vi "整合数据6.vi"(0 "Data in":u8[](array[numeric])) -> (5 "P1":u16, 6 "I1":u16, 7 "D1":u16, 8 "D2":u16, 9 "P2":u16, 10 "I2":u16)   [LabVIEW 2016]
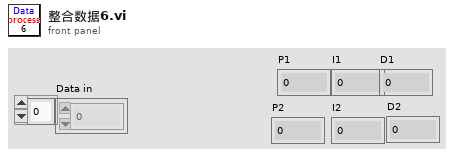
[diagram p1: front panel]
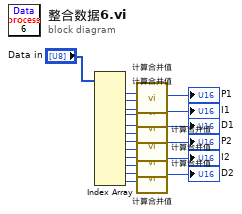
[diagram p0: block diagram]
diagram:
  n1 = Index Array(array="Data in") -> (element #1=w18:u8, element #2=w17:u8, element #3=w16:u8, element #4=w15:u8, element #5=w14:u8, element #6=w13:u8, element #7=w12:u8, element #8=w11:u8, element #9=w9:u8, element #10=w10:u8, element #11=w7:u8, element #12=w8:u8)  [unwired: 12 in]
  n2 = call "计算合并值.vi"("数值H"=w18, "数值L"=w17) -> ("合并数值"=→"P1":i16)  [unwired: 17 in]
  n3 = call "计算合并值.vi"("数值H"=w16, "数值L"=w15) -> ("合并数值"=→"I1":i16)  [unwired: 17 in]
  n4 = call "计算合并值.vi"("数值H"=w14, "数值L"=w13) -> ("合并数值"=→"D1":i16)  [unwired: 17 in]
  n5 = call "计算合并值.vi"("数值H"=w12, "数值L"=w11) -> ("合并数值"=→"P2":i16)  [unwired: 17 in]
  n6 = call "计算合并值.vi"("数值H"=w9, "数值L"=w10) -> ("合并数值"=→"I2":i16)  [unwired: 17 in]
  n7 = call "计算合并值.vi"("数值H"=w7, "数值L"=w8) -> ("合并数值"=→"D2":i16)  [unwired: 17 in]
